vi "EX 11-1 BT robot.vi"() -> ()   [LabVIEW 2011]
uses:
  <vilib>/LabVIEW Interface for Arduino/Type Defs/Board Type.ctl
  <vilib>/LabVIEW Interface for Arduino/Type Defs/Connection Type.ctl
  <vilib>/Utility/inputDevices.llb/closeJoystick.vi
  <vilib>/Utility/inputDevices.llb/joystickAcquire.vi
  <vilib>/LabVIEW Interface for Arduino/LabVIEW Interface for Arduino.lvlib
panel:
  out "Right Motor":dbl
  out "Left Motor":dbl
  in  "stop":bool
  in  "TURN Scale":dbl=100.0
  in  "FWD/REV Scale":dbl=100.0
  out "Right Y":i32
  out "Right X":i32
  out "Left Y":i32
  out "Left X":i32
  out "Right Joystick":cluster{i32[], i32[]}(graph)
  out "Left Joystick":cluster{i32[], i32[]}(graph)
  out "axis info":T1
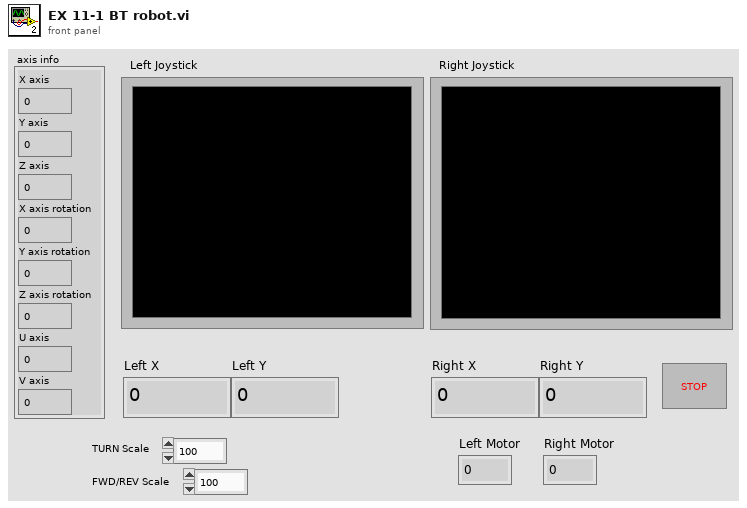
[diagram p1: front panel]
types:
  T1 = cluster{"X axis":i32, "Y axis":i32, "Z axis":i32, "X axis rotation":i32, "Y axis rotation":i32, "Z axis rotation":i32, "U axis":i32, "V axis":i32}
  T2 = cluster{"axes total":u32, "buttons total":u32, "pov total":u32, "device name":string}[]
  T3 = typedef "LabVIEW Interface for Arduino.lvlib/Board Type.ctl" = enum16{"Uno", "Dimuelanove w/Atmega 328", "Mega 2560"}
  T4 = typedef "LabVIEW Interface for Arduino.lvlib/Connection Type.ctl" = enum8{"USB / Serial", "XBEE", "BlueSmirf (Bluetooth)"}
  T5 = typedef "LabVIEW Interface for Arduino.lvlib/Arduino Resource.ctl" = cluster{"VISA resource":refnum<visa-resource-name>, "Board Type":T3, "Connection Type":enum8{"USB / Serial"}, "Bytes Per Packet (15)":u8}
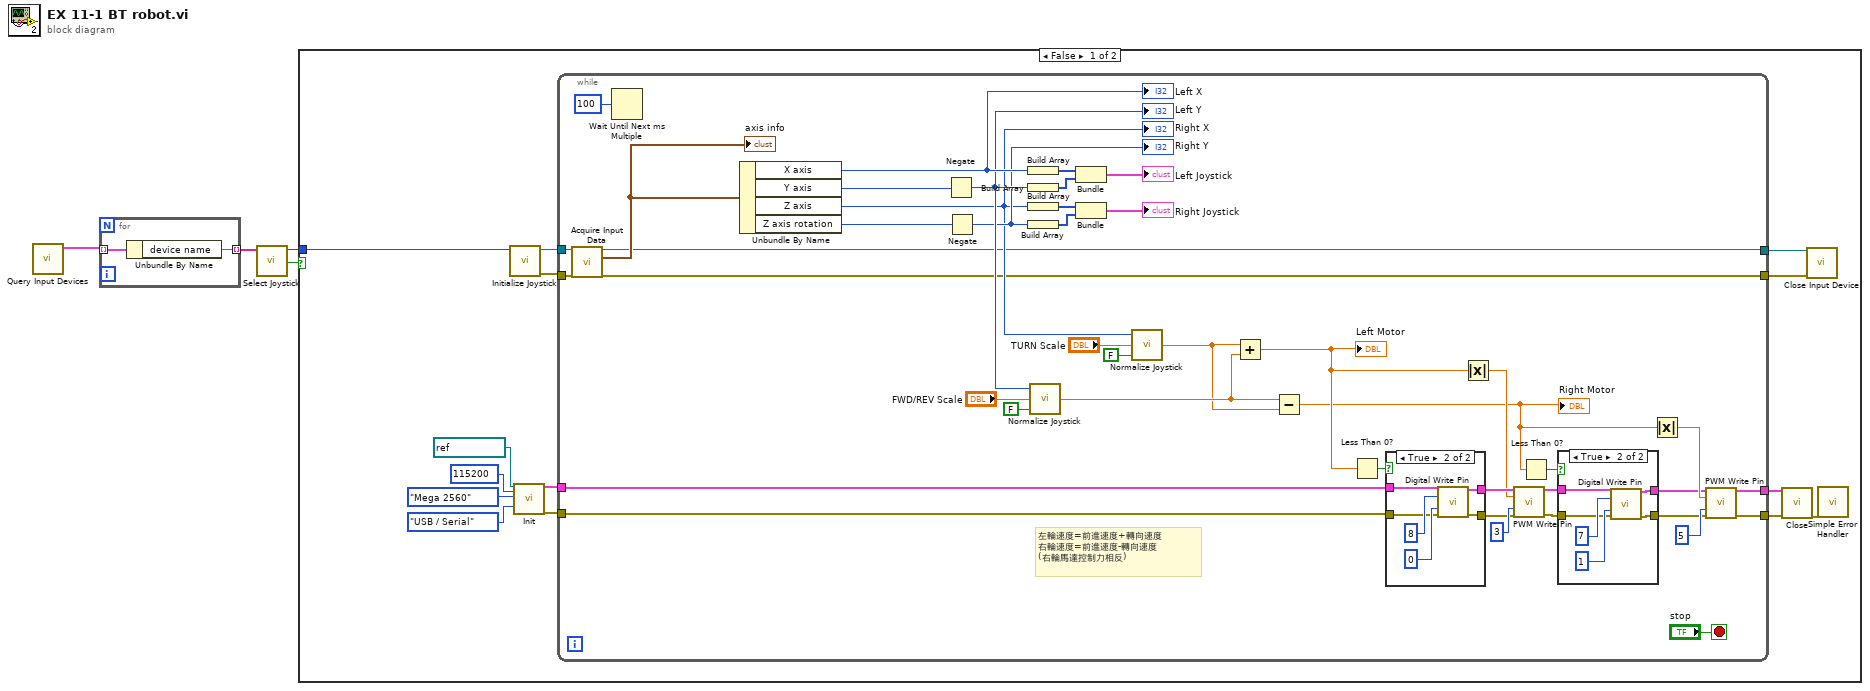
[diagram p0: block diagram]
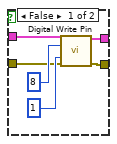
[diagram p2: hidden frame]
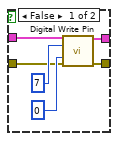
[diagram p3: hidden frame]
diagram:
  n1 = call <vilib>:"Query Input Devices.vi"() -> ("joystick info"=w4:T2)  [unwired: 8 in, 3 out]
  n2 = for {
    tunnel: w4 -> [w6] mode=indexing
    tunnel: [w5] -> w3 mode=indexing
    n3 = Unbundle By Name(w6) -> ("device name"=w5:string)
  }
  n4 = call "Select Joystick.vi"("Strings In"=w3) -> ("Cancelled?"=w2:bool, "Device out"=w1:u16)  [unwired: 9 in]
  n5 = case shown="False" w2 {
    tunnel: w1 -> [w18 _]
    frame False {
      n6 = call <vilib>:"Initialize Joystick.vi"("device index"=w18) -> ("error out"=w16:errorcluster, "device ID"=w17:refnum<k1>)  [unwired: 1 in, 8 out]
      n7 = call <vilib>:"Init.vi"("VISA resource"=refnum<visa-resource-name> "COM19", "Baud Rate (115200)"=u32 115200, "Board Type (Uno)"=Board_Type."Mega 2560", "Connection Type (USB/Serial)"=Connection_Type."USB / Serial") -> ("Arduino Resource"=w7:T5, "error out"=w15:errorcluster)  [unwired: 14 in]
      n8 = while {
        tunnel: [w43] -> w20
        tunnel: [w42] -> w19
        tunnel: w17 -> [w41]
        tunnel: w16 -> [w40]
        tunnel: w7 -> [w28]
        tunnel: w15 -> [w27]
        tunnel: [w39] -> w14
        tunnel: [w38] -> w13
        stop <- "stop" stop-if-true
        # "左輪速度=前進速度+轉向速度\n右輪速度=前進速度-轉向速度\n(右輪馬達控制力相反)"
        n9 = call-poly <vilib>:"Acquire Input Data.vi"("device ID"=w41, "error in (no error)"=w40) -> ("device ID"=w43:refnum<k1>, "axis info"=w63:T1, "error out"=w42:errorcluster)  [unwired: 15 out]
        "axis info" <- w63
        n10 = Wait Until Next ms Multiple(millisecond multiple=u32 100) -> ()  [unwired: 1 out]
        n11 = Unbundle By Name(w63) -> ("X axis"=w53:i32, "Y axis"=w61:i32, "Z axis"=w47:i32, "Z axis rotation"=w60:i32)
        "Left X" <- w53
        "Right X" <- w47
        n12 = Negate(x=w61) -> (-x=w52:i32)
        "Left Y" <- w52
        n13 = Negate(x=w60) -> (-x=w51:i32)
        "Right Y" <- w51
        n14 = Build Array(w53) -> (w59:i32[])
        n15 = Build Array(w52) -> (w58:i32[])
        n16 = Build Array(w47) -> (w56:i32[])
        n17 = Build Array(w51) -> (w55:i32[])
        n18 = call "Normalize Joystick.vi"("Reverse output?"=FALSE, "Scale"="FWD/REV Scale", "Joystick In (32767 to -32768"=w52) -> ("Output"=w45:dbl)
        n19 = Bundle(w59, w58) -> (→"Left Joystick":cluster{i32[], i32[]})  [unwired: 1 out]
        n20 = Bundle(w56, w55) -> (→"Right Joystick":cluster{i32[], i32[]})  [unwired: 1 out]
        n21 = call "Normalize Joystick.vi"("Reverse output?"=FALSE, "Scale"="TURN Scale", "Joystick In (32767 to -32768"=w47) -> ("Output"=w35:dbl)
        n22 = Add(x=w35, y=w45) -> (x+y=w24:dbl)
        "Left Motor" <- w24
        n23 = Subtract(x=w45, y=w35) -> (x-y=w21:dbl)
        "Right Motor" <- w21
        n24 = Less Than 0?(x=w24) -> (x < 0?=w23:bool)
        n25 = case shown="True" w23 {
          tunnel: [w67 w73] -> w26
          tunnel: [w66 w72] -> w25
          tunnel: w28 -> [w64 w71]
          tunnel: w27 -> [w65 w70]
          frame False {
            n26 = call <vilib>:"Digital Write Pin.vi"("Arduino Resource"=w64, "Digital I/O Pin (0)"=u8 8, "Value (0)"=u8 1, "error in"=w65) -> ("Arduino Resource"=w67:T5, "error out"=w66:errorcluster)  [unwired: 10 in]
          }
          frame True {
            n27 = call <vilib>:"Digital Write Pin.vi"("Arduino Resource"=w71, "Digital I/O Pin (0)"=u8 8, "Value (0)"=u8 0, "error in"=w70) -> ("Arduino Resource"=w73:T5, "error out"=w72:errorcluster)  [unwired: 10 in]
          }
        }
        n28 = Absolute Value(x=w24) -> (abs(x)=w22:dbl)
        n29 = call <vilib>:"PWM Write Pin.vi"("Arduino Resource"=w26, "Duty Cycle (0 - 255)"=w22, "PWM Pin (3)"=u8 3, "error in"=w25) -> ("Arduino Resource"=w32:T5, "error out"=w31:errorcluster)  [unwired: 10 in]
        n30 = Less Than 0?(x=w21) -> (x < 0?=w33:bool)
        n31 = case shown="True" w33 {
          tunnel: w32 -> [w78 w83]
          tunnel: w31 -> [w79 w82]
          tunnel: [w77 w85] -> w30
          tunnel: [w76 w84] -> w29
          frame False {
            n32 = call <vilib>:"Digital Write Pin.vi"("Arduino Resource"=w78, "Digital I/O Pin (0)"=u8 7, "Value (0)"=u8 0, "error in"=w79) -> ("Arduino Resource"=w77:T5, "error out"=w76:errorcluster)  [unwired: 10 in]
          }
          frame True {
            n33 = call <vilib>:"Digital Write Pin.vi"("Arduino Resource"=w83, "Digital I/O Pin (0)"=u8 7, "Value (0)"=u8 1, "error in"=w82) -> ("Arduino Resource"=w85:T5, "error out"=w84:errorcluster)  [unwired: 10 in]
          }
        }
        n34 = Absolute Value(x=w21) -> (abs(x)=w34:dbl)
        n35 = call <vilib>:"PWM Write Pin.vi"("Arduino Resource"=w30, "Duty Cycle (0 - 255)"=w34, "PWM Pin (3)"=u8 5, "error in"=w29) -> ("Arduino Resource"=w39:T5, "error out"=w38:errorcluster)  [unwired: 10 in]
      }
      n36 = call <vilib>:"Close.vi"("Arduino Resource"=w14, "error in"=w13) -> ("error out"=w12:errorcluster)  [unwired: 13 in]
      n37 = call-poly <vilib>:"Close Input Device.vi"("error in (no error)"=w19, "device ID"=w20) -> ()  [unwired: 9 out]
      n38 = call <vilib>:"Simple Error Handler.vi"("error in (no error)"=w12) -> ()  [unwired: 4 in, 5 out]
    }
    frame True {
    }
  }
